vi "FillFactor.vi"(11 "Depth Output":sgl[][](array[numeric])) -> (1 "Fill factor (%)":dbl, 2 "Total":i32, 3 "Filled":i32)   [LabVIEW 2017, in "libRealSense3.lvlib"]
uses:
  libRealSense3.lvlib
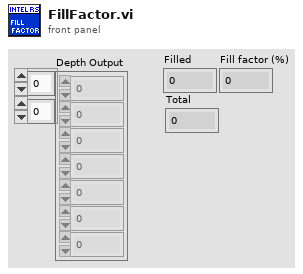
[diagram p1: front panel]
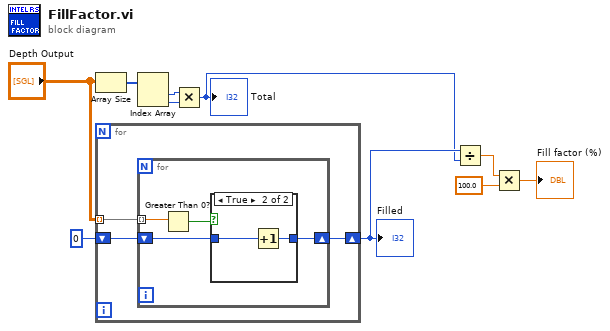
[diagram p0: block diagram]
diagram:
  n1 = Array Size(array="Depth Output") -> (size(s)=w7:i32[])
  n2 = for {
    tunnel: "Depth Output" -> [w13] mode=indexing
    shift-right: [w11] -> w5
    shift-left: 0 -> [w12]
    n3 = for {
      tunnel: w13 -> [w15] mode=indexing
      shift-right: [w16] -> w11
      shift-left: w12 -> [w17]
      n4 = Greater Than 0?(x=w15) -> (x > 0?=w14:bool)
      n5 = case shown="True" w14 {
        tunnel: w17 -> [w18 w20]
        tunnel: [w18 w19] -> w16
        frame False {
        }
        frame True {
          n6 = Increment(x=w20) -> (x+1=w19:i32)
        }
      }
    }
  }
  "Filled" <- w5
  n7 = Index Array(array=w7) -> (element #1=w8:i32, element #2=w9:i32)  [unwired: 2 in]
  n8 = Multiply(x=w8, y=w9) -> (x*y=w4:i32)
  "Total" <- w4
  n9 = Divide(x=w5, y=w4) -> (x/y=w3:dbl)
  n10 = Multiply(x=w3, y=100.0) -> (x*y=→"Fill factor (%)":dbl)
